vi "CRYSet TooBar and StatusBar.vi"(8 "StateLabel":string, 9 "variant":variant, 10 "Type":string, 11 "MainVI Ref In":refnum<vi>) -> (1 "output cluster":T1, 2 "Elapsed Ref":refnum<vi>, 3 "MainVI Ref Out":refnum<vi>)   [LabVIEW 2013]
uses:
  SubVI/CRYMain Sub Window Global.vi
  CRYSystem/Task Sequence/CRYProject Run Control Global.vi
panel:
  in  "StatusBarLabel Cluster":T2={"Label1"="Sequence", "Label2"="Category", "Label3"="Step", "Label4"="Verdict", "Numeric1"=0.0}
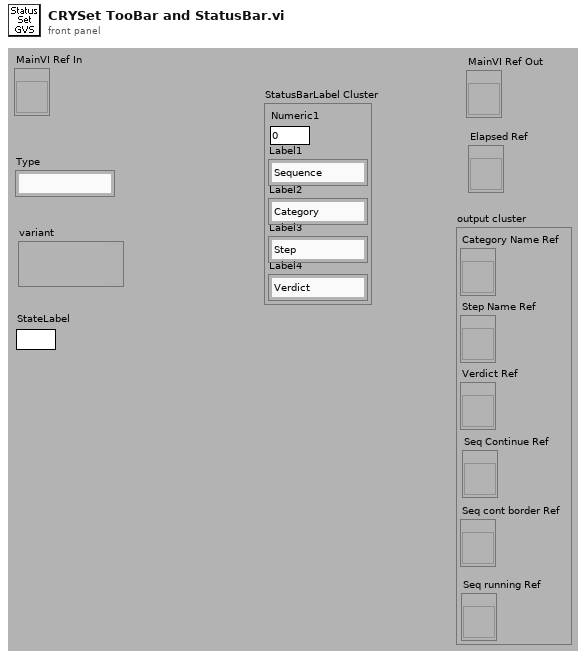
[diagram p1: front panel]
types:
  T1 = cluster{"Category Name Ref":refnum<vi>, "Step Name Ref":refnum<vi>, "Verdict Ref":refnum<vi>, "Seq Continue Ref":refnum<vi>, "Seq cont border Ref":refnum<vi>, "Seq running Ref":refnum<vi>}
  T2 = cluster{"Label1":string, "Label2":string, "Label3":string, "Label4":string, "Numeric1":dbl}
  T3 = enum8{"Enabled", "Disabled", "Disabled and Grayed Out"}
  T4 = cluster{"String Ref Out":refnum<vi>, "String Ref Out":refnum<vi>, "Boolean Ref":refnum<vi>, "Boolean Ref":refnum<vi>, "Boolean Ref":refnum<vi>, "Boolean Ref":refnum<vi>}
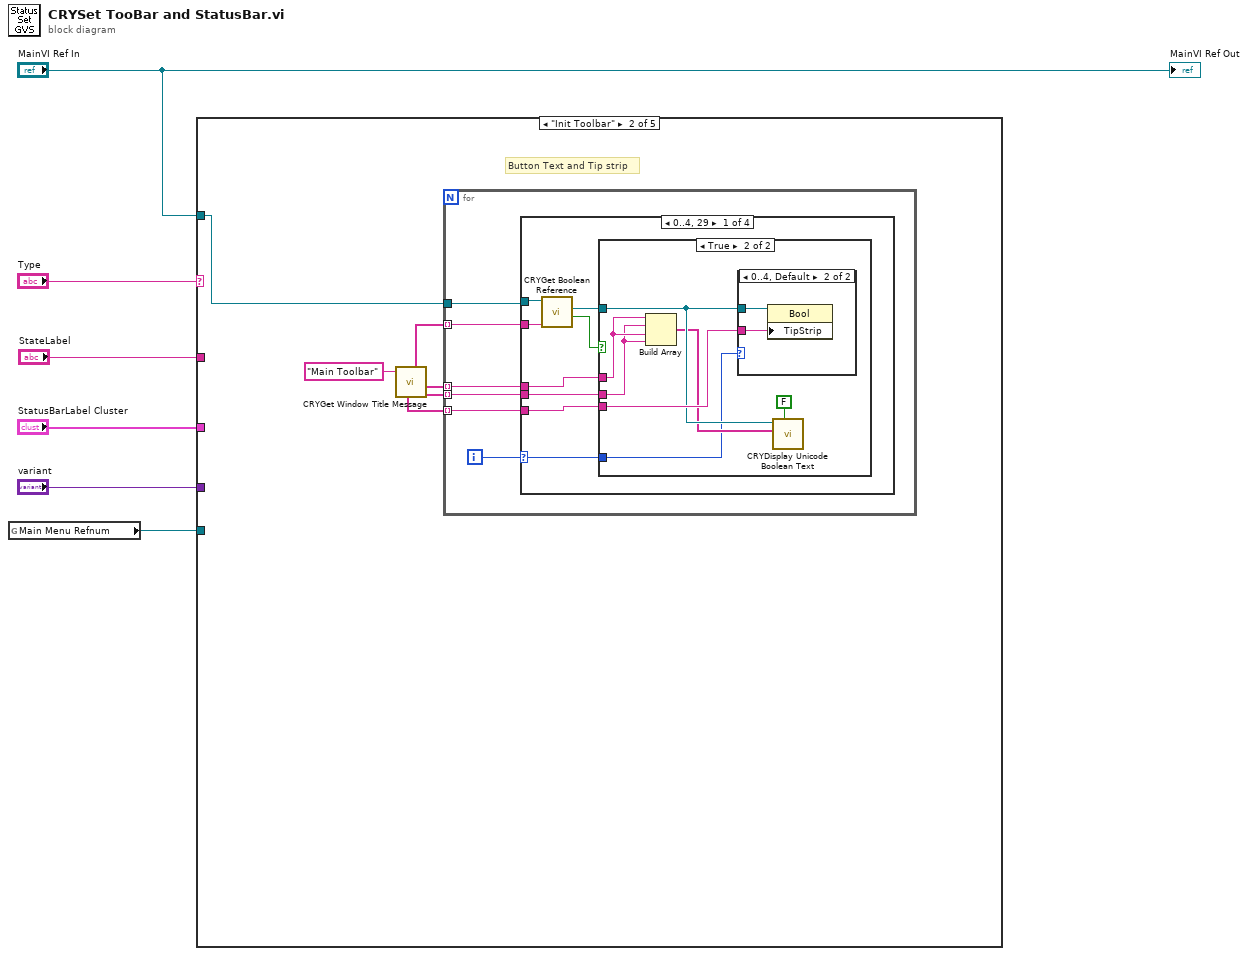
[diagram p0: block diagram]
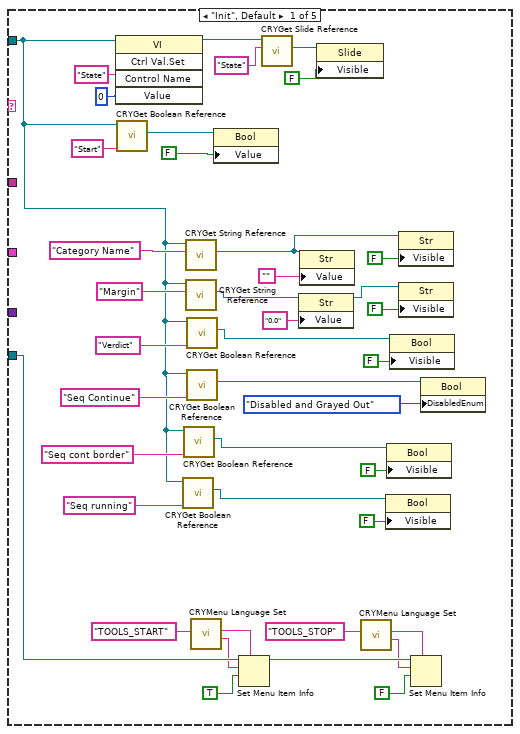
[diagram p2: hidden frame]
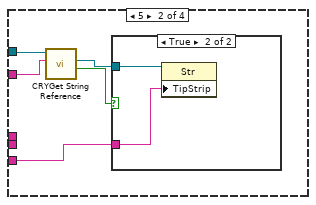
[diagram p5: hidden frame]
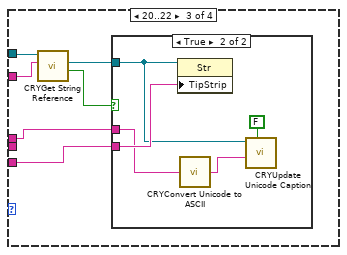
[diagram p7: hidden frame]
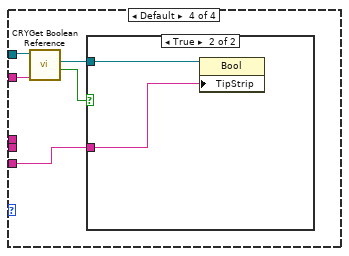
[diagram p9: hidden frame]
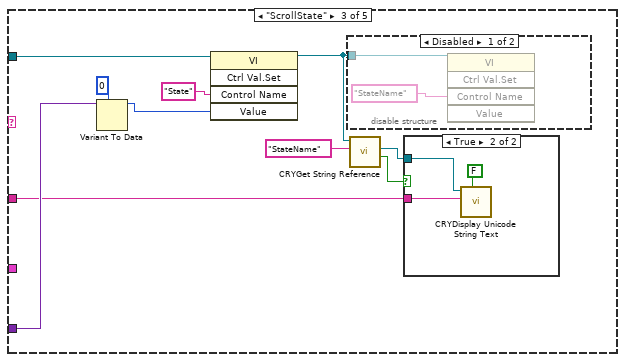
[diagram p11: hidden frame]
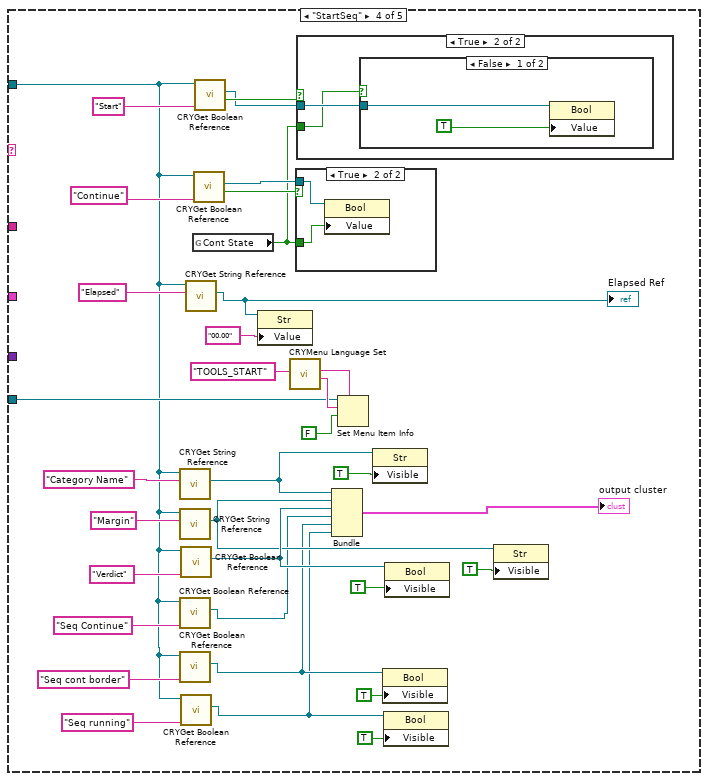
[diagram p14: hidden frame]
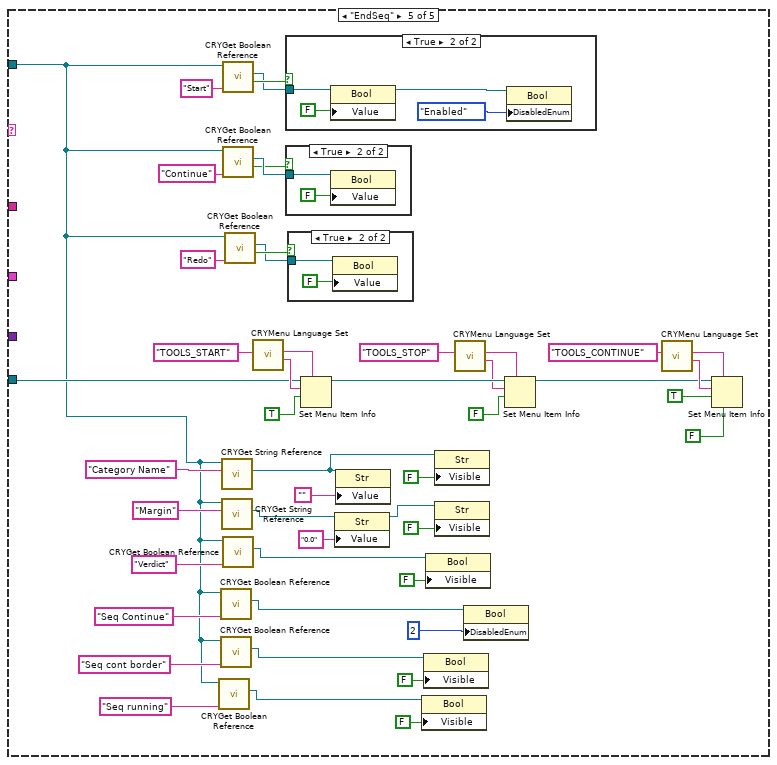
[diagram p18: hidden frame]
diagram:
  n1 = global read "CRYMain Sub Window Global.vi" "Main Menu Refnum"() -> (w2:refnum<k9>)
  n2 = case shown="\"Init Toolbar\"" "Type" {
    tunnel: "MainVI Ref In" -> [w9 w48 w110 w119 w158]
    tunnel: "variant" -> [_ _ w108 _ _]
    tunnel: "StatusBarLabel Cluster" -> [_ _ _ _ _]
    tunnel: w2 -> [w45 _ _ w146 w194]
    tunnel: "StateLabel" -> [_ _ w106 _ _]
    frame "Init", Default {
      n3 = invoke class="VI" method="Ctrl Val.Set"(reference=w9, "Control Name"="State", "Value"=0) -> (reference out=w35:refnum<vi>)  [unwired: 2 in, 4 out]
      n4 = call "CRYGet Boolean Reference.vi"("Label Name"="Start", "VI Refnum"=w9) -> ("Boolean Ref"=w43:refnum<vi>)  [unwired: 9 out]
      n5 = call "CRYGet Boolean Reference.vi"("Label Name"="Seq running", "VI Refnum"=w9) -> ("Boolean Ref"=w11:refnum<vi>)  [unwired: 9 out]
      n6 = call "CRYGet Boolean Reference.vi"("Label Name"="Seq cont border", "VI Refnum"=w9) -> ("Boolean Ref"=w16:refnum<vi>)  [unwired: 9 out]
      n7 = call "CRYGet String Reference.vi"("Label Name"="Category Name", "VI Refnum"=w9) -> ("String Ref Out"=w20:refnum<vi>)  [unwired: 7 in, 2 out]
      n8 = call "CRYGet String Reference.vi"("Label Name"="Margin", "VI Refnum"=w9) -> ("String Ref Out"=w25:refnum<vi>)  [unwired: 7 in, 2 out]
      n9 = call "CRYGet Boolean Reference.vi"("Label Name"="Verdict", "VI Refnum"=w9) -> ("Boolean Ref"=w23:refnum<vi>)  [unwired: 9 out]
      n10 = call "CRYGet Boolean Reference.vi"("Label Name"="Seq Continue", "VI Refnum"=w9) -> ("Boolean Ref"=w8:refnum<vi>)  [unwired: 9 out]
      n11 = call "CRYMenu Language Set.vi"("sID"="TOOLS_START") -> ("sMultibyte_Out"=w33:string, "sID_Out"=w34:string)  [unwired: 7 in, 2 out]
      n12 = property class="Bool"(reference=w43, "Value"=FALSE ("Visible")) -> ()  [unwired: 1 in, 2 out]
      n13 = Set Menu Item Info(7:w34, 9:TRUE ("enabled"), 10:w33, 11:w45) -> (3:w39:refnum<k9>)  [unwired: 1 in, 3 out]
      n14 = call "CRYGet Slide Reference.vi"("Label Name"="State" ("Type"), "VI Refnum"=w35) -> ("Slide Ref Out"=w38:refnum<vi>)  [unwired: 9 out]
      n15 = property class="Str"(reference=w25, "Value"="0.0") -> (reference out=w18:refnum<vi>)  [unwired: 1 in, 1 out]
      n16 = property class="Str"(reference=w20, "Value"="") -> ()  [unwired: 1 in, 2 out]
      n17 = property class="Slide"(reference=w38, "Visible"=FALSE) -> ()  [unwired: 1 in, 2 out]
      n18 = call "CRYMenu Language Set.vi"("sID"="TOOLS_STOP") -> ("sMultibyte_Out"=w31:string, "sID_Out"=w32:string)  [unwired: 7 in, 2 out]
      n19 = property class="Bool"(reference=w11, "Visible"=FALSE) -> ()  [unwired: 1 in, 2 out]
      n20 = property class="Bool"(reference=w16, "Visible"=FALSE) -> ()  [unwired: 1 in, 2 out]
      n21 = property class="Bool"(reference=w23, "Visible"=FALSE) -> ()  [unwired: 1 in, 2 out]
      n22 = property class="Str"(reference=w20, "Visible"=FALSE) -> ()  [unwired: 1 in, 2 out]
      n23 = property class="Str"(reference=w18, "Visible"=FALSE) -> ()  [unwired: 1 in, 2 out]
      n24 = Set Menu Item Info(7:w32, 9:FALSE ("enabled"), 10:w31, 11:w39) -> ()  [unwired: 1 in, 4 out]
      n25 = property class="Bool"(reference=w8, "DisabledEnum"=T3."Disabled and Grayed Out" ("Disabled")) -> ()  [unwired: 1 in, 2 out]
    }
    frame "Init Toolbar" {
      # "Button Text and Tip strip"
      n26 = call "CRYGet Window Title Message.vi"("Kind"="Main Toolbar") -> ("Control Label Off"=w49:string[], "Control Label On"=w52:string[], "Control Name"=w51:string[], "Tip Strip"=w50:string[])  [unwired: 5 in, 2 out]
      n27 = for {
        tunnel: w52 -> [w56] mode=indexing
        tunnel: w51 -> [w58] mode=indexing
        tunnel: w50 -> [w55] mode=indexing
        tunnel: w48 -> [w57]
        tunnel: w49 -> [w54] mode=indexing
        i -> [w59]
        n28 = case shown="0..4, 29" w59 {
          selector: w59 -> [w60 _ _ _]
          tunnel: w58 -> [w67 w80 w88 w99]
          tunnel: w57 -> [w66 w81 w89 w98]
          tunnel: w56 -> [w63 _ w84 _]
          tunnel: w55 -> [w64 w79 w87 w96]
          tunnel: w54 -> [w61 _ _ _]
          frame 0..4, 29 {
            n29 = call "CRYGet Boolean Reference.vi"("Label Name"=w67, "VI Refnum"=w66) -> ("Exist?"=w62:bool, "Boolean Ref"=w65:refnum<vi>)  [unwired: 8 out]
            n30 = case shown="True" w62 {
              tunnel: w65 -> [_ w71]
              tunnel: w64 -> [_ w74]
              tunnel: w63 -> [_ w73]
              tunnel: w61 -> [_ w72]
              tunnel: w60 -> [_ w68]
              frame False {
              }
              frame True {
                n31 = Build Array(w73, w72, w73, w72) -> (w70:string[])
                n32 = case shown="0..4, Default" w68 {
                  tunnel: w74 -> [_ w76]
                  tunnel: w71 -> [_ w75]
                  frame 29 {
                  }
                  frame 0..4, Default {
                    n33 = property class="Bool"(reference=w75, "TipStrip"=w76) -> ()  [unwired: 1 in, 2 out]
                  }
                }
                n34 = call "CRYDisplay Unicode Boolean Text.vi"("Interpret as Unicode (T)"=FALSE, "Boolean Texts [4]"=w70, "Boolean Reference"=w71) -> ()  [unwired: 5 in, 2 out]
              }
            }
          }
          frame 5 {
            n35 = call "CRYGet String Reference.vi"("Label Name"=w80, "VI Refnum"=w81) -> ("Find?"=w77:bool, "String Ref Out"=w78:refnum<vi>)  [unwired: 7 in, 1 out]
            n36 = case shown="True" w77 {
              tunnel: w79 -> [_ w82]
              tunnel: w78 -> [_ w83]
              frame False {
              }
              frame True {
                n37 = property class="Str"(reference=w83, "TipStrip"=w82) -> ()  [unwired: 1 in, 2 out]
              }
            }
          }
          frame 20..22 {
            n38 = call "CRYGet String Reference.vi"("Label Name"=w88, "VI Refnum"=w89) -> ("Find?"=w85:bool, "String Ref Out"=w86:refnum<vi>)  [unwired: 7 in, 1 out]
            n39 = case shown="True" w85 {
              tunnel: w87 -> [_ w94]
              tunnel: w86 -> [_ w93]
              tunnel: w84 -> [_ w91]
              frame False {
              }
              frame True {
                n40 = property class="Str"(reference=w93, "TipStrip"=w94) -> ()  [unwired: 1 in, 2 out]
                n41 = call "CRYConvert Unicode to ASCII.vi"("Unicode"=w91) -> ("ASCII"=w90:string)  [unwired: 4 in]
                n42 = call "CRYUpdate Unicode Caption.vi"("Interpret as Unicode (T)"=FALSE, "Caption"=w90, "Control Reference"=w93) -> ()  [unwired: 5 in, 2 out]
              }
            }
          }
          frame Default {
            n43 = call "CRYGet Boolean Reference.vi"("Label Name"=w99, "VI Refnum"=w98) -> ("Exist?"=w95:bool, "Boolean Ref"=w97:refnum<vi>)  [unwired: 8 out]
            n44 = case shown="True" w95 {
              tunnel: w97 -> [_ w101]
              tunnel: w96 -> [_ w100]
              frame False {
              }
              frame True {
                n45 = property class="Bool"(reference=w101, "TipStrip"=w100) -> ()  [unwired: 1 in, 2 out]
              }
            }
          }
        }
      }
    }
    frame "ScrollState" {
      n46 = Variant To Data(type=0, Variant=w108) -> (data=w107:i32)  [unwired: 1 in, 1 out]
      n47 = invoke class="VI" method="Ctrl Val.Set"(reference=w110, "Control Name"="State", "Value"=w107) -> (reference out=w105:refnum<vi>)  [unwired: 2 in, 4 out]
      n48 = disable-structure shown="Disabled" {
        disable-tunnel: w105 -> [w112 _]
        frame Disabled {
          n49 = invoke class="VI" method="Ctrl Val.Set"(reference=w112, "Control Name"="StateName") -> ()  [unwired: 2 in, 6 out]
        }
        frame Enabled {
        }
      }
      n50 = call "CRYGet String Reference.vi"("Label Name"="StateName" ("Control Name"), "VI Refnum"=w105) -> ("Find?"=w104:bool, "String Ref Out"=w103:refnum<vi>)  [unwired: 7 in, 1 out]
      n51 = case shown="True" w104 {
        tunnel: w106 -> [_ w116]
        tunnel: w103 -> [_ w115]
        frame False {
        }
        frame True {
          n52 = call "CRYDisplay Unicode String Text.vi"("Interpret as Unicode (T)"=FALSE, "String Value"=w116, "String Control Reference"=w115) -> ()  [unwired: 5 in, 2 out]
        }
      }
    }
    frame "StartSeq" {
      n53 = call "CRYGet String Reference.vi"("Label Name"="Category Name", "VI Refnum"=w119) -> ("String Ref Out"=w128:refnum<vi>)  [unwired: 7 in, 2 out]
      n54 = call "CRYGet String Reference.vi"("Label Name"="Margin", "VI Refnum"=w119) -> ("String Ref Out"=w126:refnum<vi>)  [unwired: 7 in, 2 out]
      n55 = call "CRYGet Boolean Reference.vi"("Label Name"="Seq Continue", "VI Refnum"=w119) -> ("Boolean Ref"=w117:refnum<vi>)  [unwired: 9 out]
      n56 = call "CRYGet Boolean Reference.vi"("Label Name"="Seq cont border", "VI Refnum"=w119) -> ("Boolean Ref"=w122:refnum<vi>)  [unwired: 9 out]
      n57 = call "CRYGet Boolean Reference.vi"("Label Name"="Verdict", "VI Refnum"=w119) -> ("Boolean Ref"=w130:refnum<vi>)  [unwired: 9 out]
      n58 = call "CRYGet Boolean Reference.vi"("Label Name"="Seq running", "VI Refnum"=w119) -> ("Boolean Ref"=w118:refnum<vi>)  [unwired: 9 out]
      n59 = call "CRYGet String Reference.vi"("Label Name"="Elapsed", "VI Refnum"=w119) -> ("String Ref Out"=w137:refnum<vi>)  [unwired: 7 in, 2 out]
      "Elapsed Ref" <- w137
      n60 = global read "CRYProject Run Control Global.vi" "Cont State"() -> (w136:bool)
      n61 = call "CRYGet Boolean Reference.vi"("Label Name"="Continue", "VI Refnum"=w119) -> ("Exist?"=w141:bool, "Boolean Ref"=w140:refnum<vi>)  [unwired: 8 out]
      n62 = call "CRYGet Boolean Reference.vi"("Label Name"="Start", "VI Refnum"=w119) -> ("Exist?"=w144:bool, "Boolean Ref"=w143:refnum<vi>)  [unwired: 8 out]
      n63 = property class="Str"(reference=w137, "Value"="00.00" ("Label Name")) -> ()  [unwired: 1 in, 2 out]
      n64 = call "CRYMenu Language Set.vi"("sID"="TOOLS_START") -> ("sMultibyte_Out"=w148:string, "sID_Out"=w149:string)  [unwired: 7 in, 2 out]
      n65 = case shown="True" w141 {
        tunnel: w140 -> [_ w152]
        tunnel: w136 -> [_ w151]
        frame False {
        }
        frame True {
          n66 = property class="Bool"(reference=w152, "Value"=w151) -> ()  [unwired: 1 in, 2 out]
        }
      }
      n67 = case shown="True" w144 {
        tunnel: w143 -> [_ w154]
        tunnel: w136 -> [_ w153]
        frame False {
        }
        frame True {
          n68 = case shown="False" w153 {
            tunnel: w154 -> [w156 _]
            frame False {
              n69 = property class="Bool"(reference=w156, "Value"=TRUE ("Cont State")) -> ()  [unwired: 1 in, 2 out]
            }
            frame True {
            }
          }
        }
      }
      n70 = Bundle("String Ref Out"=w128, "String Ref Out"=w126, "Boolean Ref"=w130, "Boolean Ref"=w117, "Boolean Ref"=w122, "Boolean Ref"=w118) -> (→"output cluster":T4)  [unwired: 1 in]
      n71 = Set Menu Item Info(7:w149, 9:FALSE ("enabled"), 10:w148, 11:w146) -> ()  [unwired: 1 in, 4 out]
      n72 = property class="Str"(reference=w128, "Visible"=TRUE) -> ()  [unwired: 1 in, 2 out]
      n73 = property class="Bool"(reference=w122, "Visible"=TRUE) -> ()  [unwired: 1 in, 2 out]
      n74 = property class="Bool"(reference=w118, "Visible"=TRUE) -> ()  [unwired: 1 in, 2 out]
      n75 = property class="Bool"(reference=w130, "Visible"=TRUE) -> ()  [unwired: 1 in, 2 out]
      n76 = property class="Str"(reference=w126, "Visible"=TRUE) -> ()  [unwired: 1 in, 2 out]
    }
    frame "EndSeq" {
      n77 = call "CRYGet Boolean Reference.vi"("Label Name"="Seq running", "VI Refnum"=w158) -> ("Boolean Ref"=w159:refnum<vi>)  [unwired: 9 out]
      n78 = call "CRYGet Boolean Reference.vi"("Label Name"="Seq Continue", "VI Refnum"=w158) -> ("Boolean Ref"=w162:refnum<vi>)  [unwired: 9 out]
      n79 = call "CRYGet Boolean Reference.vi"("Label Name"="Seq cont border", "VI Refnum"=w158) -> ("Boolean Ref"=w166:refnum<vi>)  [unwired: 9 out]
      n80 = call "CRYGet String Reference.vi"("Label Name"="Category Name", "VI Refnum"=w158) -> ("String Ref Out"=w170:refnum<vi>)  [unwired: 7 in, 2 out]
      n81 = call "CRYGet String Reference.vi"("Label Name"="Margin", "VI Refnum"=w158) -> ("String Ref Out"=w175:refnum<vi>)  [unwired: 7 in, 2 out]
      n82 = call "CRYGet Boolean Reference.vi"("Label Name"="Start", "VI Refnum"=w158) -> ("Exist?"=w185:bool, "Boolean Ref"=w184:refnum<vi>)  [unwired: 8 out]
      n83 = call "CRYGet Boolean Reference.vi"("Label Name"="Continue", "VI Refnum"=w158) -> ("Exist?"=w186:bool, "Boolean Ref"=w187:refnum<vi>)  [unwired: 8 out]
      n84 = call "CRYGet Boolean Reference.vi"("Label Name"="Verdict", "VI Refnum"=w158) -> ("Boolean Ref"=w173:refnum<vi>)  [unwired: 9 out]
      n85 = call "CRYGet Boolean Reference.vi"("Label Name"="Redo", "VI Refnum"=w158) -> ("Exist?"=w180:bool, "Boolean Ref"=w179:refnum<vi>)  [unwired: 8 out]
      n86 = call "CRYMenu Language Set.vi"("sID"="TOOLS_START") -> ("sMultibyte_Out"=w199:string, "sID_Out"=w200:string)  [unwired: 7 in, 2 out]
      n87 = case shown="True" w185 {
        tunnel: w184 -> [_ w210]
        frame False {
        }
        frame True {
          n88 = property class="Bool"(reference=w210, "Value"=FALSE) -> (reference out=w209:refnum<vi>)  [unwired: 1 in, 1 out]
          n89 = property class="Bool"(reference=w209, "DisabledEnum"=T3."Enabled" ("Disabled")) -> ()  [unwired: 1 in, 2 out]
        }
      }
      n90 = case shown="True" w186 {
        tunnel: w187 -> [_ w206]
        frame False {
        }
        frame True {
          n91 = property class="Bool"(reference=w206, "Value"=FALSE) -> ()  [unwired: 1 in, 2 out]
        }
      }
      n92 = case shown="True" w180 {
        tunnel: w179 -> [_ w204]
        frame False {
        }
        frame True {
          n93 = property class="Bool"(reference=w204, "Value"=FALSE) -> ()  [unwired: 1 in, 2 out]
        }
      }
      n94 = Set Menu Item Info(7:w200, 9:TRUE ("enabled"), 10:w199, 11:w194) -> (3:w201:refnum<k9>)  [unwired: 1 in, 3 out]
      n95 = property class="Str"(reference=w175, "Value"="0.0") -> (reference out=w168:refnum<vi>)  [unwired: 1 in, 1 out]
      n96 = property class="Str"(reference=w170, "Value"="") -> ()  [unwired: 1 in, 2 out]
      n97 = property class="Bool"(reference=w159, "Visible"=FALSE) -> ()  [unwired: 1 in, 2 out]
      n98 = property class="Bool"(reference=w166, "Visible"=FALSE) -> ()  [unwired: 1 in, 2 out]
      n99 = property class="Bool"(reference=w173, "Visible"=FALSE) -> ()  [unwired: 1 in, 2 out]
      n100 = property class="Str"(reference=w170, "Visible"=FALSE) -> ()  [unwired: 1 in, 2 out]
      n101 = property class="Str"(reference=w168, "Visible"=FALSE) -> ()  [unwired: 1 in, 2 out]
      n102 = call "CRYMenu Language Set.vi"("sID"="TOOLS_STOP") -> ("sMultibyte_Out"=w197:string, "sID_Out"=w198:string)  [unwired: 7 in, 2 out]
      n103 = property class="Bool"(reference=w162, "DisabledEnum"=2) -> ()  [unwired: 1 in, 2 out]
      n104 = Set Menu Item Info(7:w198, 9:FALSE ("enabled"), 10:w197, 11:w201) -> (3:w189:refnum<k9>)  [unwired: 1 in, 3 out]
      n105 = call "CRYMenu Language Set.vi"("sID"="TOOLS_CONTINUE") -> ("sMultibyte_Out"=w192:string, "sID_Out"=w191:string)  [unwired: 7 in, 2 out]
      n106 = Set Menu Item Info(6:FALSE ("enabled"), 7:w191, 9:TRUE ("enabled"), 10:w192, 11:w189) -> ()  [unwired: 1 in, 3 out]
    }
  }
  "MainVI Ref Out" <- "MainVI Ref In"
